vi "WILT Panel Dryer Details.vi"(0 "Dryer In":T4 {"Night Cycle Count" format="%04d"; "Day Cycle Count" format="%04d"}, 1 "FileName":path caption="Sample Datafilename", 9 "Test State":T2) -> (4 "Dryer Details Out":T3, 6 "New Filenames":bool, 8 "Updated":bool, 10 "Audit Alert Out":bool)   [LabVIEW 2016]
uses:
  Type Definitions/WILT Dryer.ctl
  Type Definitions/WILT Dryer Details.ctl
  Type Definitions/WILT Agilent Channel Definition.ctl
  Type Definitions/WILT DAQ Data.ctl
  Type Definitions/WILT Dryer Test State.ctl
  Globals/Globals Wilt.vi
panel:
  in  "Audit Alert Button":bool
  in  "Return":bool
  out "Time":dbl[](array[numeric])
  out "Cycle Count":dbl[](array[numeric])
  in  "Tab Control":T1(tab)
  out "Dryer Details":T3
  out "Total Cycle Count":i32
  out "Station Number":string
  out "Status Color":u32(colorbox)
  out "Bad Com Count":i32
  out "Com Port":u8
  out "Boolean":bool
  out "Audit Alert":bool
  out "Sample Plot":cluster{dbl[], dbl[]}[](graph)
  out "Current Cycle Count":dbl
  out "I(L1),I(L2),Trmb,V.V2":dbl[][](array[numeric])
  out "Cycle Count 2":dbl[](array[numeric])
  out "Completion time":dbl[](array[numeric])
  out "L1max":dbl[](array[numeric])
  out "L2max":dbl[](array[numeric])
  out "Tmax":dbl[](array[numeric])
  out "History Plot":cluster{dbl, dbl}[](graph)
  out "Serial Com Array":cluster{dbl, string}[](array[cluster]) {"?" format="%<%H:%M:%S>t"}
  out "Voltage 2":dbl[](array[numeric])
  out "Voltage":dbl[](array[numeric])
  out "Trmb":dbl[](array[numeric])
  out "L2":dbl[](array[numeric])
  out "L1":dbl[](array[numeric])
  out "Sample Record":string[][](array[string])
  out "all rows":string[][](array[string])
  in  "Read Sample Record(t, CC, Tc, \nASCII, Status, L1,L2,Trmb,V{,V2,SW} )":string[][](array[string])
  in  "Update":bool
  # "Day"
  # "Night"
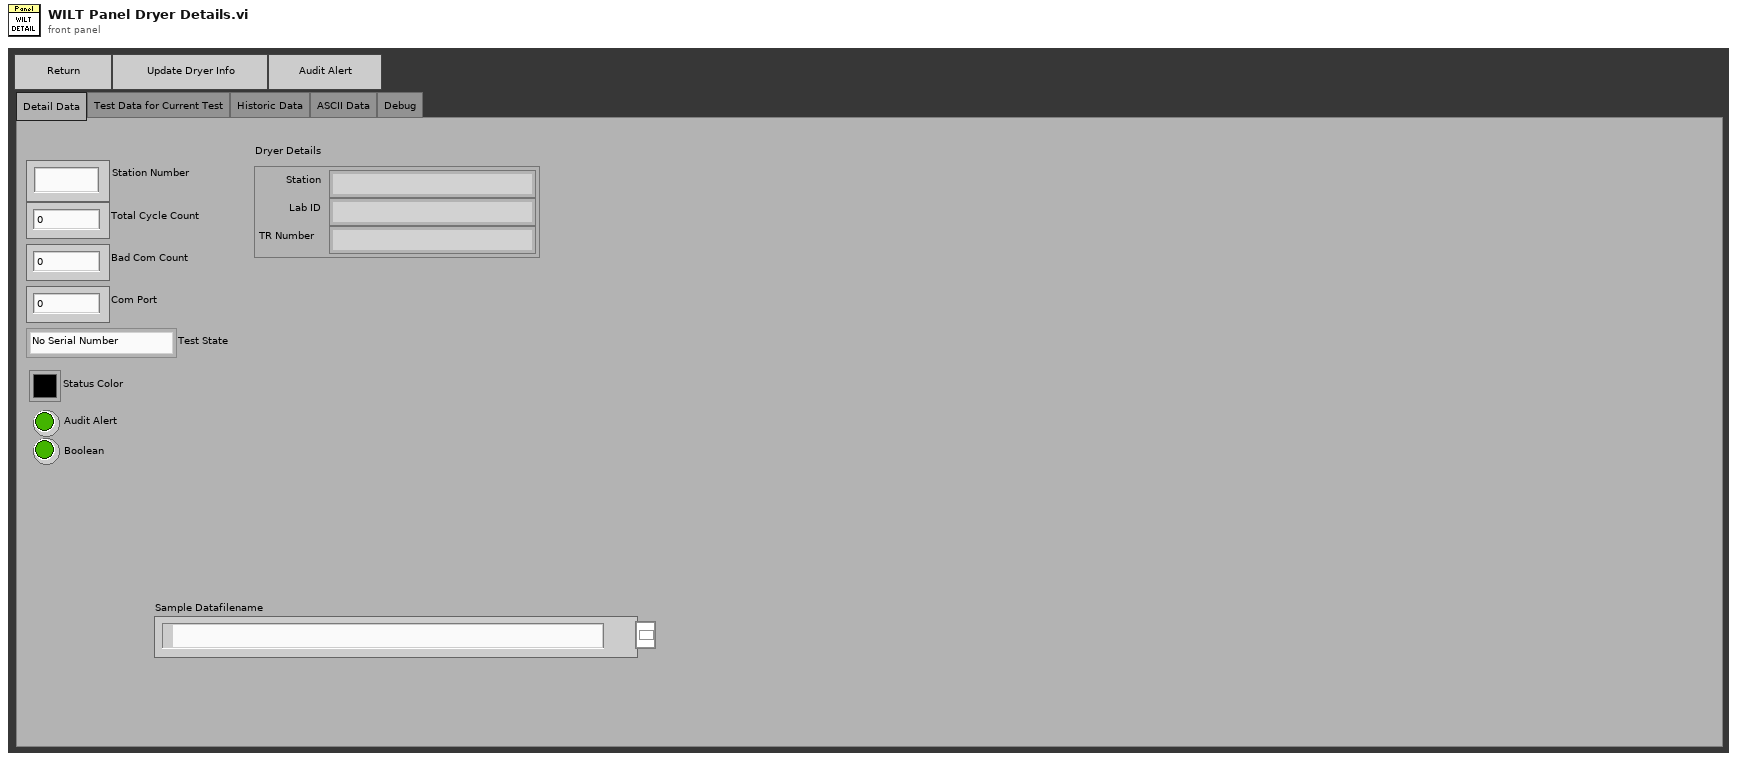
[diagram p1: front panel]
types:
  T1 = enum32{"Detail Data", "Test Data for Current Test", "Historic Data", "ASCII Data", "Debug"}
  T2 = typedef "WILT Dryer Test State.ctl" = enum16{"No Serial Number", "Waiting for Dryer To Start", "Drying Clothes", "Water Injection 1 (On)", "Water Injection 1 Timer", "Water Injection 1 (Off)", "Pause Dryer", "Sending Start Stop CMD", "Pause Dryer 2", "Sending Start Stop CMD 2", "Drying Clothes 2", "Water Injection 2 (On)", "Water Injection 2 Timer", "Water Injection 2 (Off)", "Drying Clothes 3", "Cooling Down", "Sending Start Stop CMD 3", "Increment Cycle"}
  T3 = typedef "WILT Dryer Details.ctl" = cluster{"Station":string, "Lab ID":string, "TR Number":string}
  T4 = typedef "WILT Dryer.ctl" = cluster{"Lab ID":string, "Day Cycle Count":i32, "Station Label":string, "Dryer Details":T3, "Status Color":u32, "Invisible Button":bool, "Night Cycle Count":i32, "Station Index":i32, "Cycle Index":string, "Audit Alert":bool, "Agilent Channel Definition":T5, "DAQ Data":T6}
  T5 = typedef "WILT Agilent Channel Definition.ctl" = cluster{"Channel":string, "Station":string, "Label":string, "Agilent Station":string, "Data":dbl}
  T6 = typedef "WILT DAQ Data.ctl" = cluster{"L1 Current":dbl, "L2 Current":dbl, "Temperature  Deg F (TC)":dbl, "Volts":dbl, "Volts (208)":dbl, "SW (208)":dbl}
  T7 = enum16{"Read 2D Array", "Write 2D Array", "Write/Append 1D Array"}
  T8 = cluster{"FileName":path, "New File Info":bool, "Dryer In":T4, "Read Sample Record(t, CC, Tc, \nASCII, Status, L1,L2,Trmb,V{,V2,SW} )":string[][], "Audit Alert":bool, "Updated":bool}
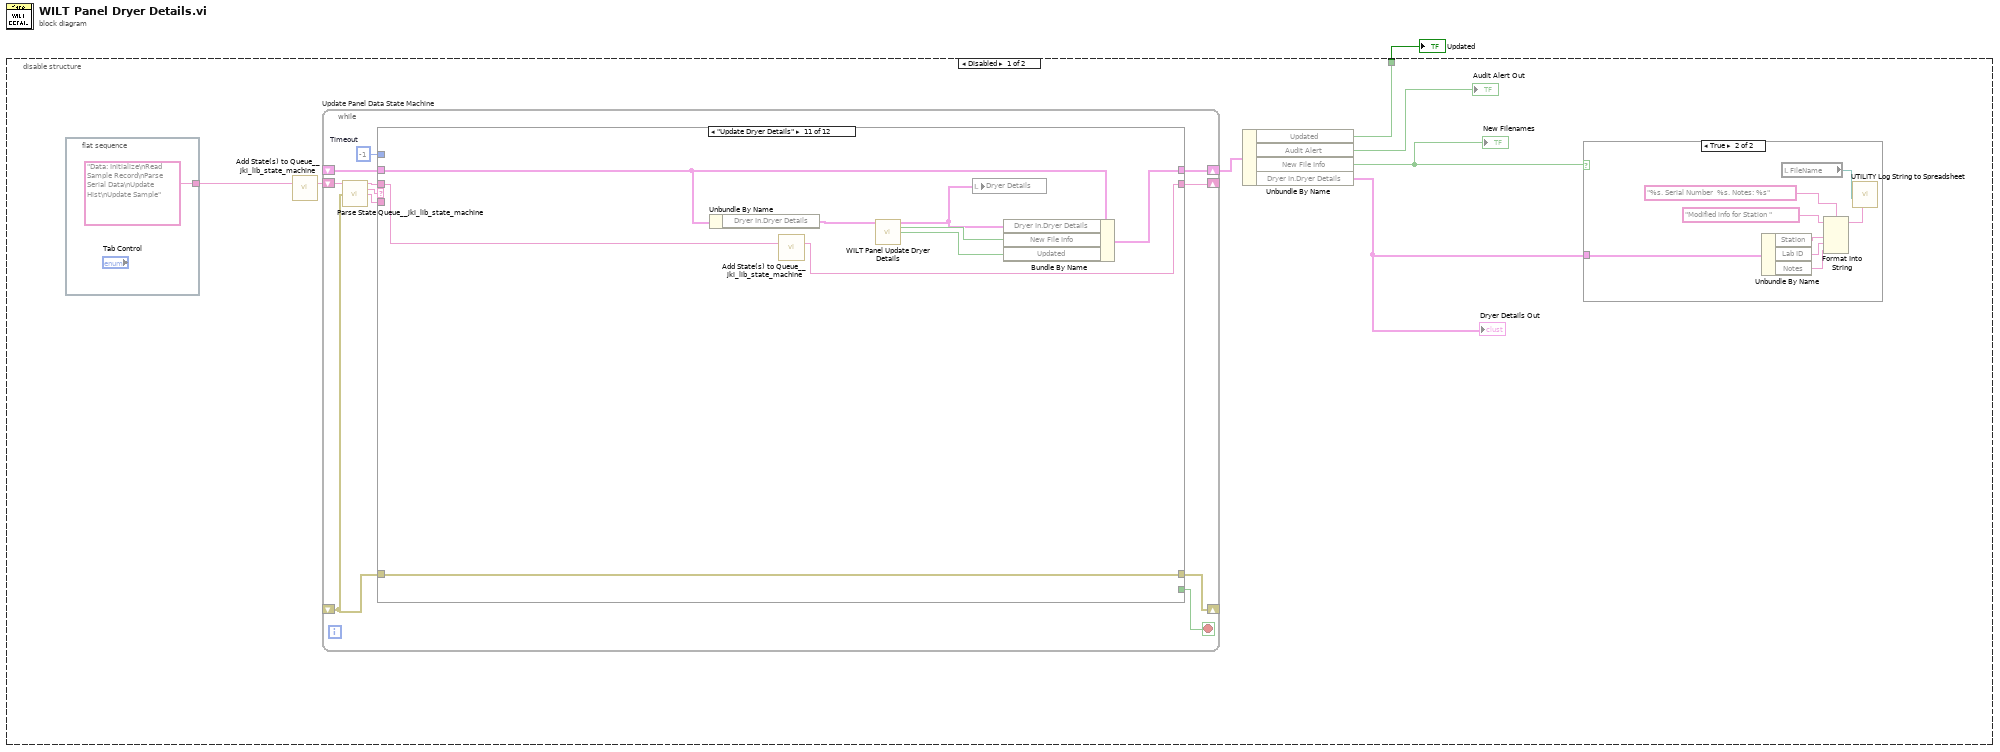
[diagram p0: block diagram]
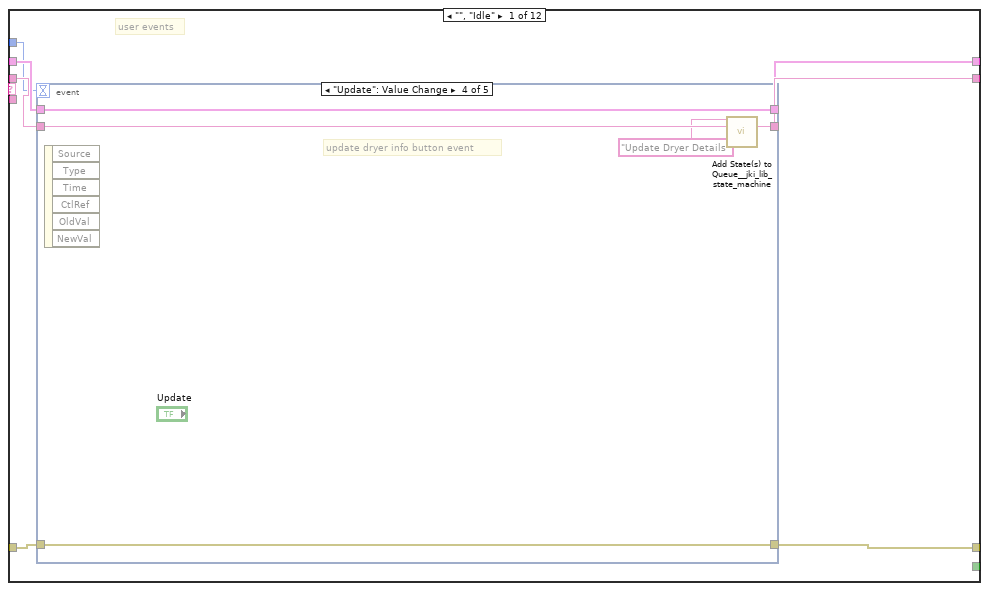
[diagram p2: hidden frame]
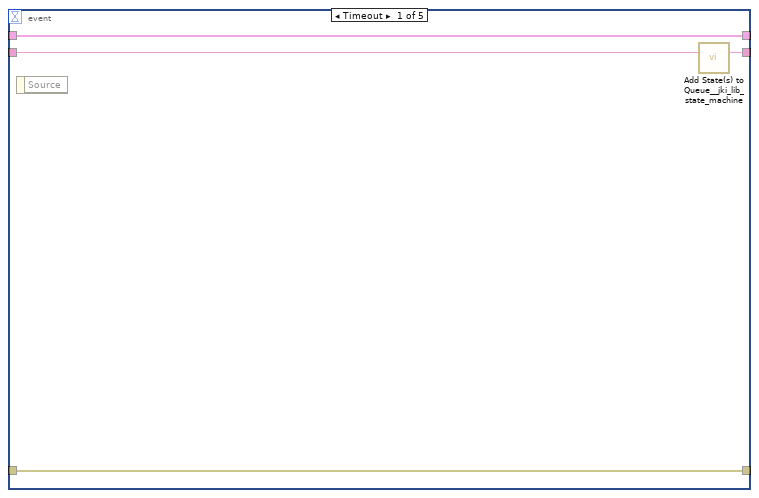
[diagram p3: hidden frame]
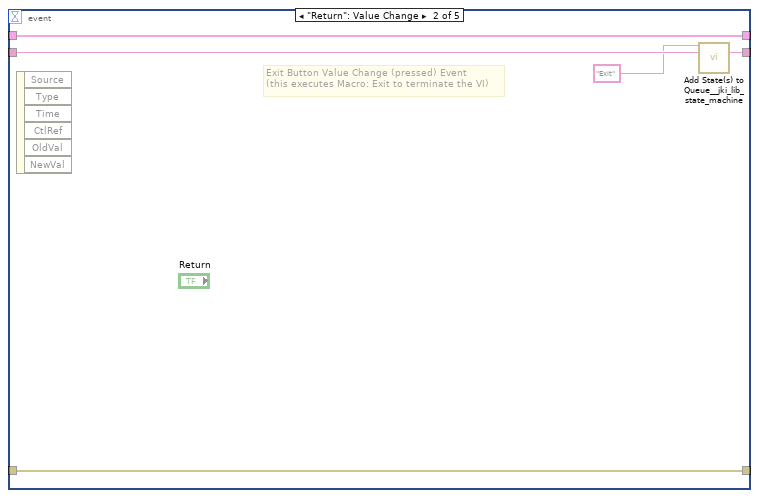
[diagram p4: hidden frame]
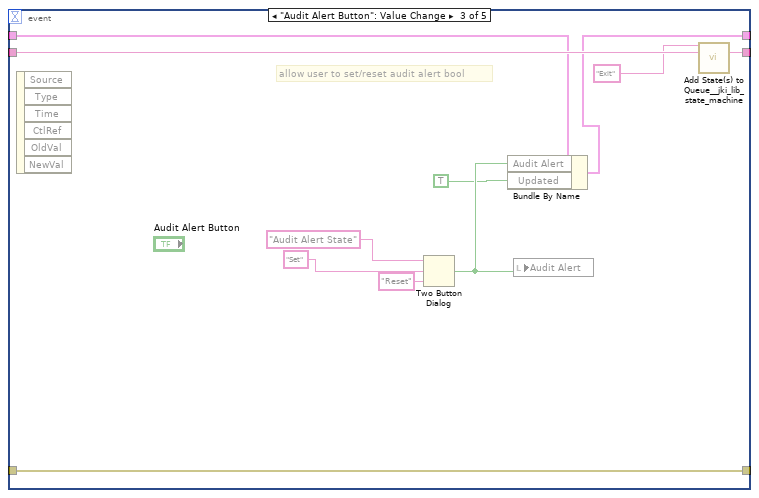
[diagram p5: hidden frame]
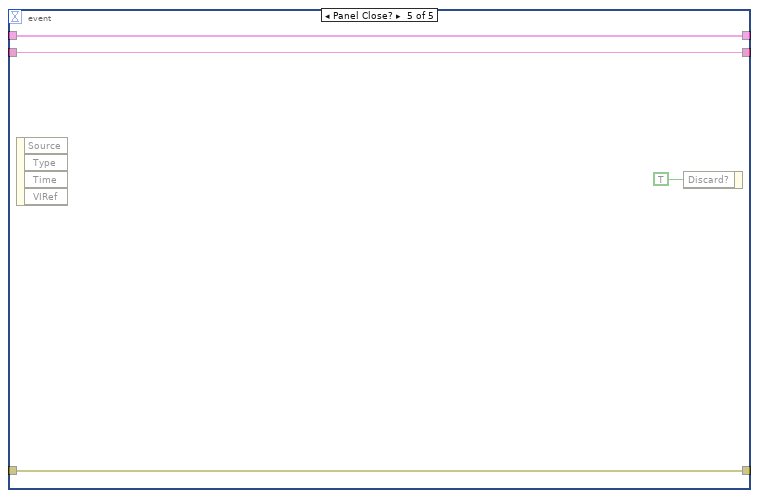
[diagram p6: hidden frame]
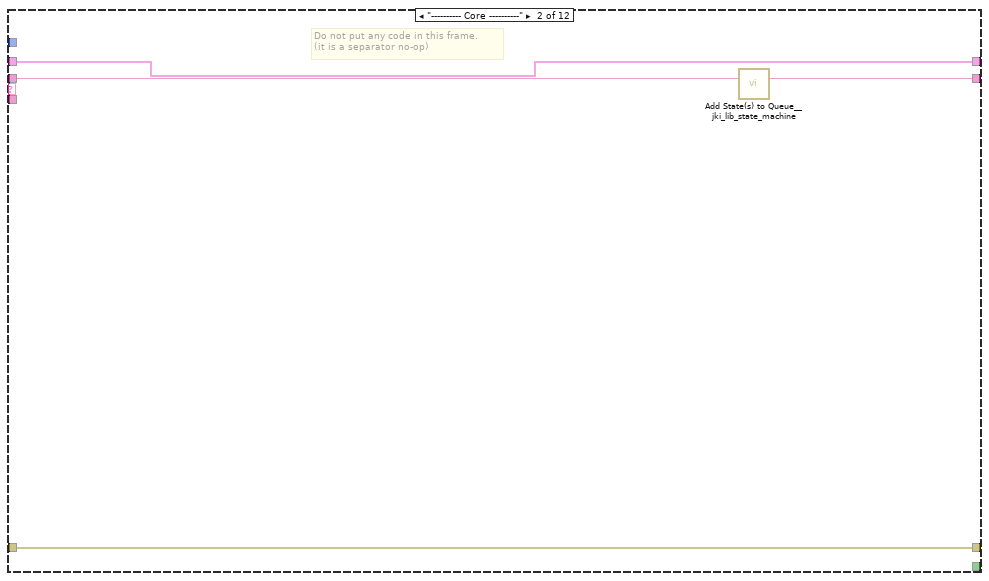
[diagram p7: hidden frame]
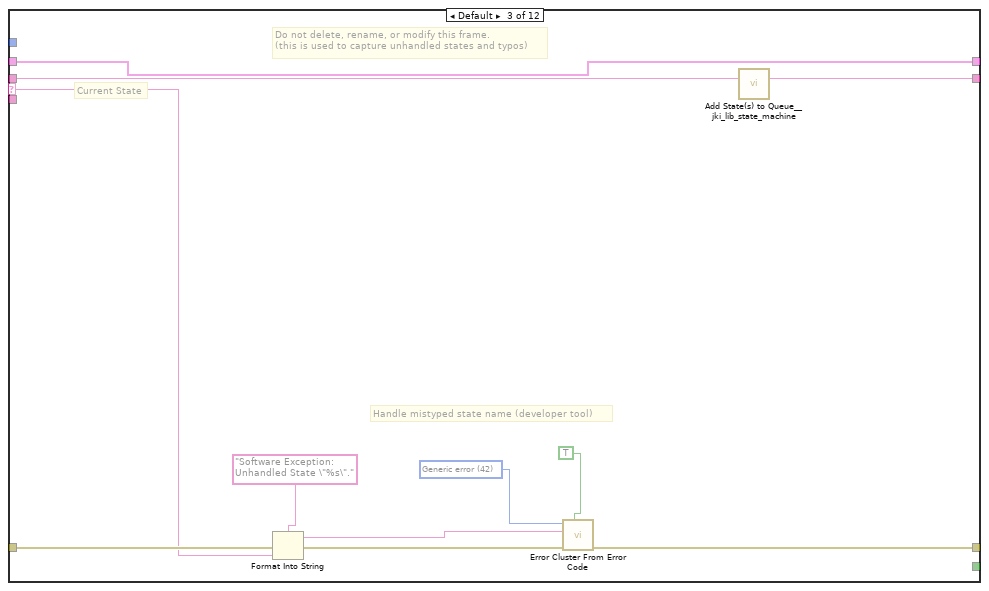
[diagram p8: hidden frame]
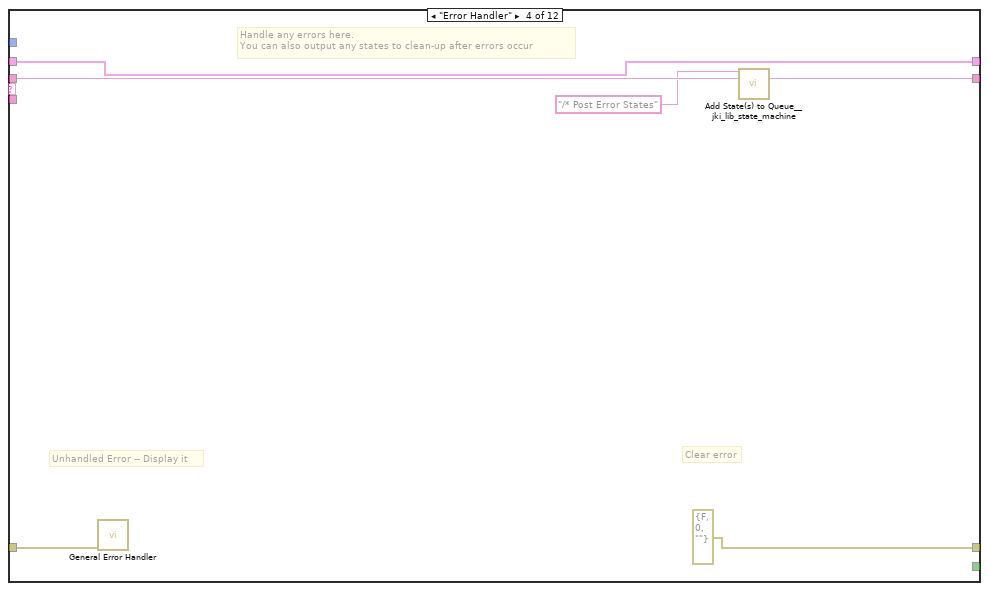
[diagram p9: hidden frame]
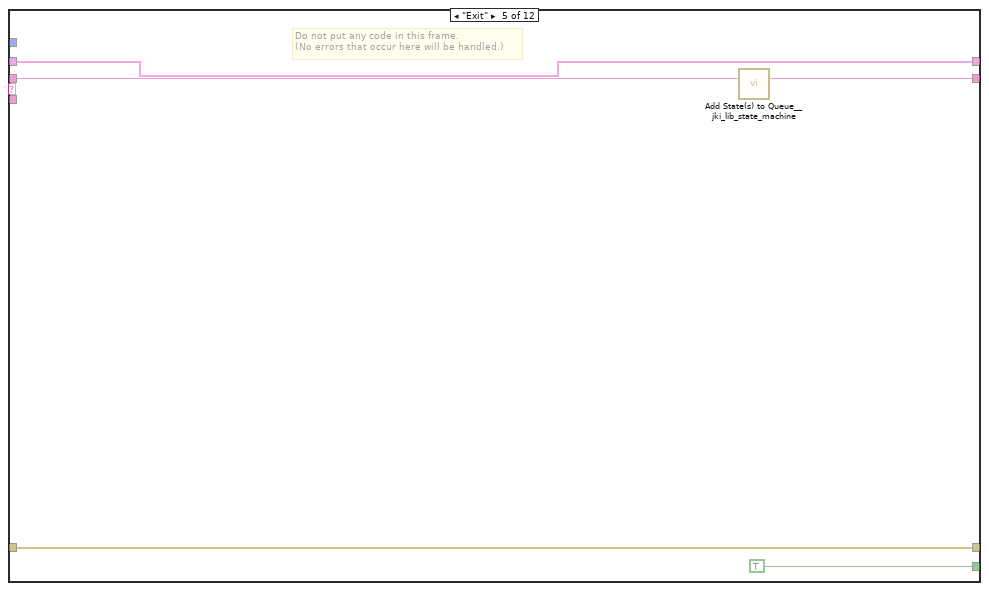
[diagram p10: hidden frame]
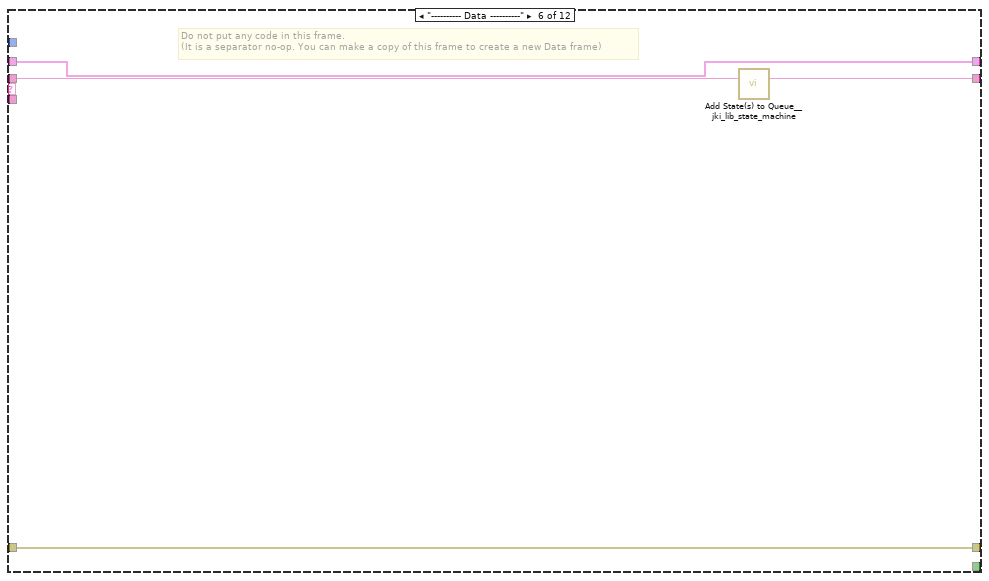
[diagram p11: hidden frame]
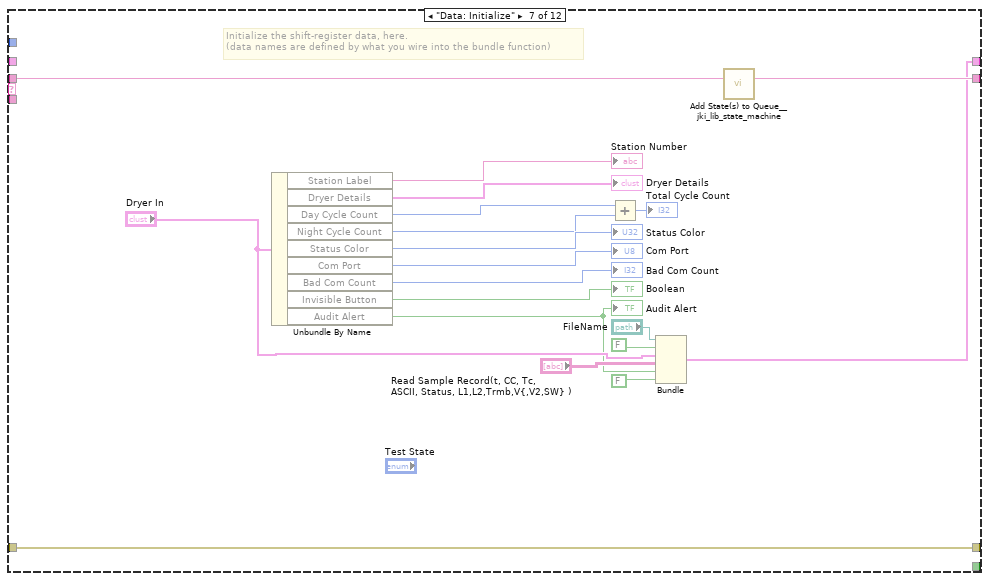
[diagram p12: hidden frame]
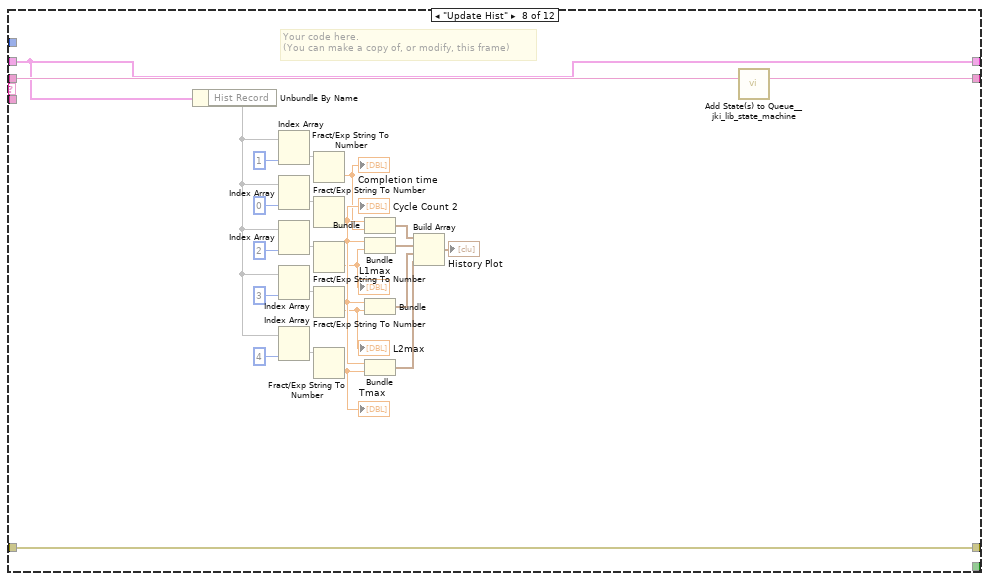
[diagram p13: hidden frame]
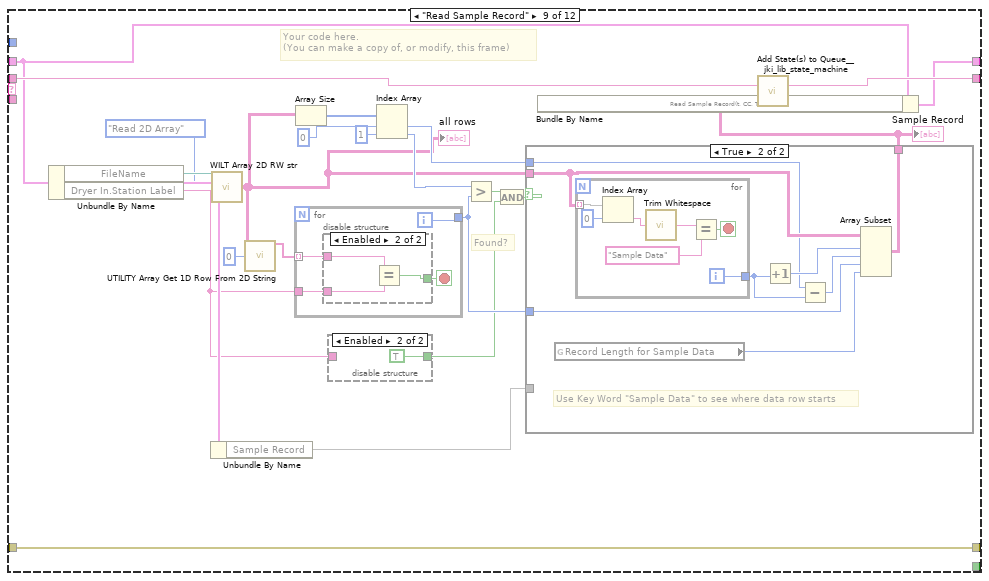
[diagram p14: hidden frame]
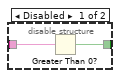
[diagram p15: hidden frame]
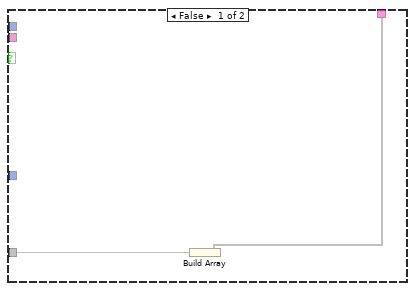
[diagram p16: hidden frame]
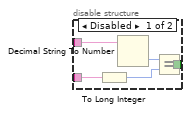
[diagram p17: hidden frame]
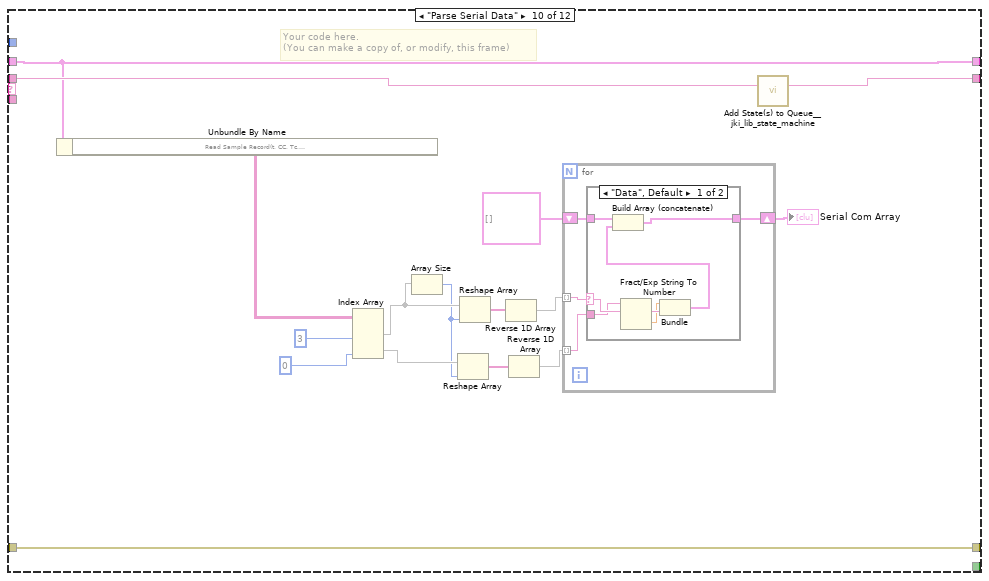
[diagram p18: hidden frame]
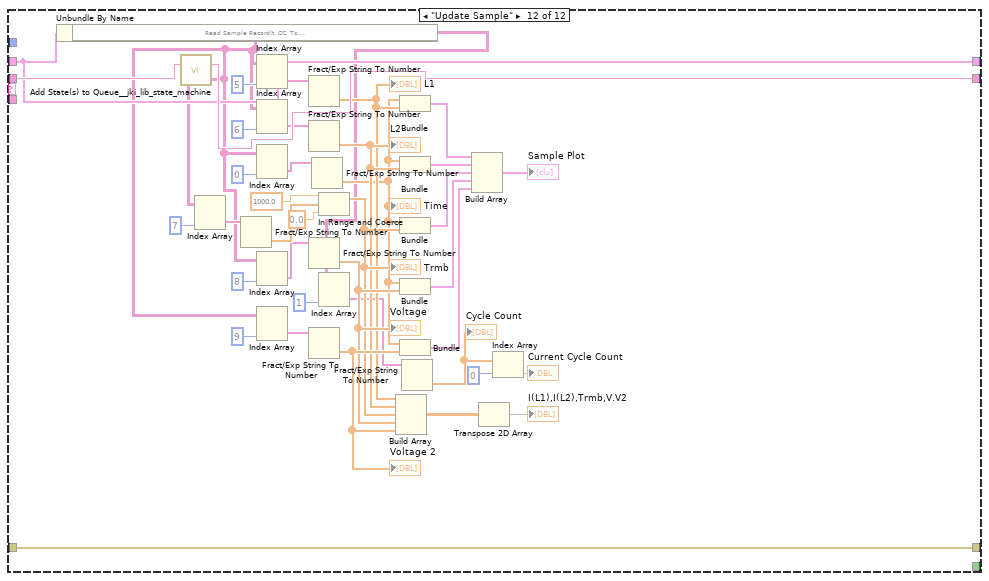
[diagram p20: hidden frame]
diagram:
  n1 = disable-structure shown="Disabled" {
    disable-tunnel: [w2 _] -> w1
    frame Disabled {
      n2 = flat-sequence {
        tunnel: ["Data: Initialize\nRead Sample Record\nParse Serial Data\nUpdate Hist\nUpdate Sample"] -> w7
        frame #0 {
        }
      }
      n3 = call <vilib>:"Add State(s) to Queue__jki_lib_state_machine.vi"("State(s) in (\"\")"=w7) -> ("States Out"=w8:string)  [unwired: 14 in]
      n4 = while "Update Panel Data State Machine" {
        shift-right: [w13] -> w6
        shift-left: _ -> [w12]
        shift-right: [w16] -> _
        shift-left: _ -> [w10]
        shift-right: [w15] -> _
        shift-left: w8 -> [w17]
        stop <- w14 stop-if-true
        w11 = -1  # Timeout
        n5 = call <vilib>:"Parse State Queue__jki_lib_state_machine.vi"("State Queue"=w17, "Error In (no error)"=w10) -> ("Remaining States"=w19:string, "Current State"=w20:string, "Arguments"=w18:string)  [unwired: 11 in]
        n6 = case shown="\"Update Dryer Details\"" w20 {
          selector: w20 -> [_ _ w61 _ _ _ _ _ _ _ _ _]
          tunnel: w19 -> [w27 w60 w65 w77 w82 w86 w105 w130 w152 w200 w220 w259]
          tunnel: w18 -> [_ _ _ _ _ _ _ _ _ _ _ _]
          tunnel: w12 -> [w25 w57 w63 w74 w80 w83 _ w107 w146 w197 w216 w222]
          tunnel: [w24 w58 w67 errorcluster {"status"=FALSE, "code"=0, "source"=""} ("error out") w79 w84 w102 w128 w150 w198 w218 w257] -> w16
          tunnel: w10 -> [w23 w58 w66 w73 w79 w84 w102 w128 w150 w198 w218 w257]
          tunnel: [w26 w59 w64 w76 w81 w85 w104 w129 w151 w199 w219 w258] -> w15
          tunnel: [_ _ _ _ TRUE _ _ _ _ _ _ _] -> w14
          tunnel: [w22 w57 w63 w74 w80 w83 w103 w107 w145 w197 w215 w222] -> w13
          tunnel: w11 -> [w21 _ _ _ _ _ _ _ _ _ _ _]
          frame "", "Idle" {
            # "user events"
            n7 = event shown="[3] \"Update\": Value Change" {
              selector: _ -> [_ _ _ _ _]
              dyn-events: _ -> [_ _ _ _ _]
              timeout: w21 -> [_ _ _ _ _]
              tunnel: w27 -> [w31 w36 w47 w52 w55]
              tunnel: [w30 w35 w46 w51 w55] -> w26
              tunnel: w25 -> [w28 w33 w40 w49 w56]
              tunnel: [w29 w34 w45 w50 w53] -> w24
              tunnel: w23 -> [w29 w34 w45 w50 w53]
              tunnel: [w28 w33 w39 w49 w56] -> w22
              event Timeout {
                n8 = event-data() -> ()  [unwired: 1 in, 1 out]
                n9 = call <vilib>:"Add State(s) to Queue__jki_lib_state_machine.vi"("State(s) in (\"\")"=w31) -> ("States Out"=w30:string)  [unwired: 14 in]
              }
              event "Return": Value Change {
                # "Exit Button Value Change (pressed) Event\n(this executes Macro: Exit to terminate the VI)"
                n10 = event-data() -> ()  [unwired: 1 in, 6 out]
                n11 = call <vilib>:"Add State(s) to Queue__jki_lib_state_machine.vi"("State(s) in Front (\"\")"="Exit", "State(s) in (\"\")"=w36) -> ("States Out"=w35:string)  [unwired: 13 in]
              }
              event "Audit Alert Button": Value Change {
                # "allow user to set/reset audit alert bool"
                n12 = event-data() -> ()  [unwired: 1 in, 6 out]
                n13 = Two Button Dialog(message="Audit Alert State", 1:"Reset" ("F button name (\"Cancel\")"), 2:"Set" ("T button name (\"OK\")")) -> (T button?=w38:bool)
                n14 = Bundle By Name(cluster=w40, "Audit Alert"=w38, "Updated"=TRUE) -> (w39:T8)
                n15 = local write "Audit Alert"(w38) -> ()
                n16 = call <vilib>:"Add State(s) to Queue__jki_lib_state_machine.vi"("State(s) in Front (\"\")"="Exit", "State(s) in (\"\")"=w47) -> ("States Out"=w46:string)  [unwired: 13 in]
              }
              event "Update": Value Change {
                # "update dryer info button event"
                n17 = event-data() -> ()  [unwired: 1 in, 6 out]
                n18 = call <vilib>:"Add State(s) to Queue__jki_lib_state_machine.vi"("State(s) in Front (\"\")"="Update Dryer Details", "State(s) in (\"\")"=w52) -> ("States Out"=w51:string)  [unwired: 13 in]
              }
              event Panel Close? {
                n19 = event-data() -> ()  [unwired: 1 in, 4 out]
                n20 = event-data("Discard?"=TRUE) -> ()  [unwired: 1 in, 1 out]
              }
            }
          }
          frame "---------- Core ----------" {
            # "Do not put any code in this frame.\n(it is a separator no-op)"
            n21 = call <vilib>:"Add State(s) to Queue__jki_lib_state_machine.vi"("State(s) in (\"\")"=w60) -> ("States Out"=w59:string)  [unwired: 14 in]
          }
          frame Default {
            w70 = 42 items=["No error", "Argument error", "Memory is full", "Out of zone", "End of file", "File already open", "Generic file I/O error", "File not found", "File permission error", "Disk is full", "Duplicate path", "Too many files open", "System feature not enabled", "Resource file not found", "Cannot add resource", "Resource not found", "Image not found", "Image memory error", "Pen does not exist", "Config type invalid", "Config token not found", "Config parse error", "Config memory error", "Bad external code format", "Bad external code offset", "External code not present", "Null window", "Destroy window error", "Null menu", "Print aborted", "Bad print record", "Print driver error", "Windows error during printing", "Memory error during printing", "Print dialog error", "Generic print error", "Invalid device refnum", "Device not found", "Device parameter error", "Device unit error", "Cannot open device", "Device call aborted", "Generic error", "Cancelled by user", "Object ID too low", "Object ID too high", "Object not in heap", "Unknown heap", "Unknown object (invalid DefProc)", "Unknown object (DefProc not in table)", "Message out of range", "Invalid (null) method", "Unknown message", "Manager call not supported", "Bad address", "Network operation in progress", "Network operation timed out", "Connection is busy", "Network attribute not supported", "Network error", "Address in use", "System out of memory", "Connection aborted", "Connection refused", "Not connected", "Already connected", "Connection closed", "Initialization error (interapplication manager)", "Bad occurrence", "Wait on unbound occurrence handler", "Occurrence queue overflow", "Datalog type conflict", "Unused", "Unrecognized type (interapplication manager)", "Memory corrupt", "Failed to make temporary DLL", "Old CIN version", "Drag socket not found", "Failed to load drop-object", "Failed to register OLE object", "Failed to release OLE object", "Format specifier type mismatch", "Unknown format specifier", "Too few format specifiers", "Too many format specifiers", "Scan failed", "Newer CIN version", "Error converting to variant", "Runtime menu error", "Password tampered", "Variant attribute not found", "Incompatible variant data type", "Event data is not available", "Event Store is not present", "Occurrence is not found", "Event Queue is not created", "Event info is not available", "Refnum passed is NULL", "Error retrieving Class GUID", "Error retrieving CoClass GUID", "Error retrieving TypeLib GUID.", "Bad built application magic bytes.", "Specific driver is different from the specific driver associated with the Logical Name.", "There is no session opened to the class driver.", "Max Error", "MAX - Error with config objects", "MAX - Error loading configuration", "MAX - Group not supported"]
            # "Current State"
            # "Do not delete, rename, or modify this frame.\n(this is used to capture unhandled states and typos)"
            # "Handle mistyped state name (developer tool)"
            n22 = Format Into String(format string="Software Exception: Unhandled State \"%s\"." ("message"), error in=w66, w61) -> (resulting string=w69:string, error out=w68:errorcluster)  [unwired: 1 in]
            n23 = call <vilib>:"Error Cluster From Error Code.vi"("show call chain? (False)"=TRUE, "error in (no error)"=w68, "error message (\"\")"=w69, "error code (0)"=w70) -> ("error out"=w67:errorcluster)  [unwired: 5 in]
            n24 = call <vilib>:"Add State(s) to Queue__jki_lib_state_machine.vi"("State(s) in (\"\")"=w65) -> ("States Out"=w64:string)  [unwired: 14 in]
          }
          frame "Error Handler" {
            # "Unhandled Error -- Display it"
            # "Handle any errors here.\nYou can also output any states to clean-up after errors occur"
            # "Clear error"
            n25 = call <vilib>:"General Error Handler.vi"("error in (no error)"=w73) -> ()  [unwired: 10 in, 5 out]
            n26 = call <vilib>:"Add State(s) to Queue__jki_lib_state_machine.vi"("State(s) in Front (\"\")"="/* Post Error States", "State(s) in (\"\")"=w77) -> ("States Out"=w76:string)  [unwired: 13 in]
          }
          frame "Exit" {
            # "Do not put any code in this frame.\n(No errors that occur here will be handled.)"
            n27 = call <vilib>:"Add State(s) to Queue__jki_lib_state_machine.vi"("State(s) in (\"\")"=w82) -> ("States Out"=w81:string)  [unwired: 14 in]
          }
          frame "---------- Data ----------" {
            # "Do not put any code in this frame.\n(It is a separator no-op. You can make a copy of this frame to create a new Data frame)"
            n28 = call <vilib>:"Add State(s) to Queue__jki_lib_state_machine.vi"("State(s) in (\"\")"=w86) -> ("States Out"=w85:string)  [unwired: 14 in]
          }
          frame "Data: Initialize" {
            # "Initialize the shift-register data, here.\n(data names are defined by what you wire into the bundle function)"
            n29 = Unbundle By Name("Dryer In") -> ("Station Label"=→"Station Number":string, "Dryer Details"=→"Dryer Details":T3, "Day Cycle Count"=w91:i32, "Night Cycle Count"=w90:i32, "Status Color"=→"Status Color":u32, "Com Port"=→"Com Port":u8, "Bad Com Count"=→"Bad Com Count":i32, "Invisible Button"=→"Boolean":bool, "Audit Alert"=w88:bool)
            "Audit Alert" <- w88
            n30 = Add(x=w91, y=w90) -> (x+y=→"Total Cycle Count":i32)
            n31 = Bundle("FileName"="FileName", "New File Info"=FALSE, "Dryer In"="Dryer In", "Read Sample Record(t, CC, Tc, \nASCII, Status, L1,L2,Trmb,V{,V2,SW} )"="Read Sample Record(t, CC, Tc, \nASCII, Status, L1,L2,Trmb,V{,V2,SW} )", "Audit Alert"=w88, "Updated"=FALSE) -> (w103:T8)  [unwired: 1 in]
            n32 = call <vilib>:"Add State(s) to Queue__jki_lib_state_machine.vi"("State(s) in (\"\")"=w105) -> ("States Out"=w104:string)  [unwired: 14 in]
          }
          frame "Update Hist" {
            # "Your code here.\n(You can make a copy of, or modify, this frame)"
            n33 = Unbundle By Name(w107) -> ("Hist Record"=w106)
            n34 = Index Array(array=w106, index (col)=1 ("disabled index (col)")) -> (element=w110)  [unwired: 1 in]
            n35 = Index Array(array=w106, index (col)=0 ("disabled index (col)")) -> (element=w108)  [unwired: 1 in]
            n36 = Index Array(array=w106, index (col)=2 ("disabled index (col)")) -> (element=w111)  [unwired: 1 in]
            n37 = Index Array(array=w106, index (col)=3 ("disabled index (col)")) -> (element=w115)  [unwired: 1 in]
            n38 = Index Array(array=w106, index (col)=4 ("disabled index (col)")) -> (element=w124)  [unwired: 1 in]
            n39 = Fract/Exp String To Number(string=w110) -> (number=w116:dbl)  [unwired: 3 in, 1 out]
            "Completion time" <- w116
            n40 = Fract/Exp String To Number(string=w108) -> (number=w126:dbl)  [unwired: 3 in, 1 out]
            "Cycle Count 2" <- w126
            n41 = Fract/Exp String To Number(string=w111) -> (number=w117:dbl)  [unwired: 3 in, 1 out]
            "L1max" <- w117
            n42 = Fract/Exp String To Number(string=w115) -> (number=w118:dbl)  [unwired: 3 in, 1 out]
            "L2max" <- w118
            n43 = Fract/Exp String To Number(string=w124) -> (number=w125:dbl)  [unwired: 3 in, 1 out]
            "Tmax" <- w125
            n44 = Bundle(w126, w116) -> (w120:cluster{dbl, dbl})  [unwired: 1 out]
            n45 = Bundle(w126, w117) -> (w121:cluster{dbl, dbl})  [unwired: 1 out]
            n46 = Bundle(w126, w118) -> (w122:cluster{dbl, dbl})  [unwired: 1 out]
            n47 = Bundle(w126, w125) -> (w127:cluster{dbl, dbl})  [unwired: 1 out]
            n48 = Build Array(w120, w121, w122, w127) -> (→"History Plot":cluster{dbl, dbl}[])
            n49 = call <vilib>:"Add State(s) to Queue__jki_lib_state_machine.vi"("State(s) in (\"\")"=w130) -> ("States Out"=w129:string)  [unwired: 14 in]
          }
          frame "Read Sample Record" {
            # "Found?"
            # "Your code here.\n(You can make a copy of, or modify, this frame)"
            n50 = Unbundle By Name(w146) -> ("FileName"=w133:path, "Dryer In.Station Label"=w141:string)
            n51 = Unbundle By Name(w146) -> ("Sample Record"=w139)
            n52 = call "WILT Array 2D RW str.vi"("file path (dialog if empty)"=w133, "Write/Read"=T7."Read 2D Array") -> ("Read all rows"=w132:string[][])  [unwired: 13 in]
            "all rows" <- w132
            n53 = call "UTILITY Array Get 1D Row From 2D String.vi"("all rows"=w132, "row index"=0) -> ("row"=w136:string[])  [unwired: 13 in]
            n54 = for {
              tunnel: w136 -> [w176] mode=indexing
              tunnel: w141 -> [w175]
              tunnel: [w173] -> w147
              i -> [w173]
              stop <- w174 stop-if-true
              n55 = disable-structure shown="Enabled" {
                disable-tunnel: w176 -> [w181 w183]
                disable-tunnel: w175 -> [w179 w184]
                disable-tunnel: [w177 w182] -> w174
                frame Disabled {
                  n56 = To Long Integer(number=w179) -> (32bit integer=w178:i32)
                  n57 = Decimal String To Number(string=w181) -> (number=w180:i32)  [unwired: 2 in, 1 out]
                  n58 = Equal?(x=w180, y=w178) -> (x = y?=w177:bool)
                }
                frame Enabled {
                  n59 = Equal?(x=w183, y=w184) -> (x = y?=w182:bool)
                }
              }
            }
            n60 = Array Size(array=w132) -> (size(s)=w149:i32[])
            n61 = disable-structure shown="Enabled" {
              disable-tunnel: w141 -> [w154 _]
              disable-tunnel: [w153 TRUE] -> w140
              frame Disabled {
                n62 = Greater Than 0?(x=w154) -> (x > 0?=w153:bool)
              }
              frame Enabled {
              }
            }
            n63 = Index Array(array=w149, index #1=0 ("index"), index #2=1 ("index")) -> (element #1=w134:i32, element #2=w137:i32)
            n64 = Greater?(x=w137, y=w147) -> (0:w143:bool)
            n65 = And(x=w143, y=w140) -> (x .and. y?=w142:bool)
            n66 = case shown="True" w142 {
              tunnel: w132 -> [_ w164]
              tunnel: w147 -> [_ w163]
              tunnel: [w156 w162] -> w144
              tunnel: w139 -> [w157 _]
              tunnel: w134 -> [_ w159]
              frame False {
                n67 = Build Array(w157) -> (w156:void[])
              }
              frame True {
                # "Use Key Word \"Sample Data\" to see where data row starts"
                n68 = global read "Globals Wilt.vi" "Record Length for Sample Data"() -> (w161:i32)
                n69 = for {
                  tunnel: w164 -> [w172] mode=indexing
                  tunnel: [w169] -> w158
                  i -> [w169]
                  stop <- w168 stop-if-true
                  n70 = Index Array(array=w172, index=0) -> (element=w167:string)
                  n71 = call <vilib>:"Trim Whitespace.vi"("string"=w167) -> ("trimmed string"=w166:string)  [unwired: 1 in]
                  n72 = Equal?(x=w166, y="Sample Data") -> (x = y?=w168:bool)
                }
                n73 = Increment(x=w158) -> (x+1=w165:i32)
                n74 = Subtract(x=w159, y=w158) -> (x-y=w160:i32)
                n75 = Array Subset(array=w164, index (row)=w165, length (row)=w160, index (col)=w163, length (col)=w161) -> (w162:string[][])
              }
            }
            "Sample Record" <- w144
            n76 = Bundle By Name(cluster=w146, "Read Sample Record(t, CC, Tc, \nASCII, Status, L1,L2,Trmb,V{,V2,SW} )"=w144) -> (w145:T8)
            n77 = call <vilib>:"Add State(s) to Queue__jki_lib_state_machine.vi"("State(s) in (\"\")"=w152) -> ("States Out"=w151:string)  [unwired: 14 in]
          }
          frame "Parse Serial Data" {
            # "Your code here.\n(You can make a copy of, or modify, this frame)"
            n78 = Unbundle By Name(w197) -> ("Read Sample Record(t, CC, Tc, \nASCII, Status, L1,L2,Trmb,V{,V2,SW} )"=w187:string[][])
            n79 = Index Array(array=w187, index (col) #1=3 ("disabled index (col)"), index (col) #2=0 ("index (col)")) -> (element #1=w186:string[], element #2=w193:string[])  [unwired: 2 in]
            n80 = Array Size(array=w186) -> (size(s)=w185:i32)
            n81 = Reshape Array(w193, w185) -> (w192:string[])
            n82 = Reshape Array(w186, w185) -> (w195:string[])
            n83 = Reverse 1D Array(array=w195) -> (reversed array=w191:string[])
            n84 = Reverse 1D Array(array=w192) -> (reversed array=w190:string[])
            n85 = for {
              tunnel: w191 -> [w204] mode=indexing
              tunnel: w190 -> [w203] mode=indexing
              shift-right: [w202] -> w189
              shift-left: cluster{dbl, string}[] [] -> [w201]
              n86 = case shown="\"Data\", Default" w204 {
                selector: w204 -> [w210 _]
                tunnel: w203 -> [w209 _]
                tunnel: [w207 w211] -> w202
                tunnel: w201 -> [w206 w211]
                frame "Data", Default {
                  n87 = Fract/Exp String To Number(string=w209) -> (number=w205:dbl)  [unwired: 3 in, 1 out]
                  n88 = Bundle(w205, w210) -> (w208:cluster{dbl, string})  [unwired: 1 in]
                  n89 = Build Array (concatenate)(w206, w208) -> (w207:cluster{dbl, string}[])
                }
                frame "" {
                }
              }
            }
            "Serial Com Array" <- w189
            n90 = call <vilib>:"Add State(s) to Queue__jki_lib_state_machine.vi"("State(s) in (\"\")"=w200) -> ("States Out"=w199:string)  [unwired: 14 in]
          }
          frame "Update Dryer Details" {
            n91 = Unbundle By Name(w216) -> ("Dryer In.Dryer Details"=w217:T3)
            n92 = call <vilib>:"Add State(s) to Queue__jki_lib_state_machine.vi"("State(s) in (\"\")"=w220) -> ("States Out"=w219:string)  [unwired: 14 in]
            n93 = call "WILT Panel Update Dryer Details.vi"("Dryer Details In"=w217) -> ("Dryer Details Out"=w213:T3, "New Filenames"=w214:bool, "Updated"=w212:bool)  [unwired: 12 in]
            n94 = local write "Dryer Details"(w213) -> ()
            n95 = Bundle By Name(cluster=w216, "Dryer In.Dryer Details"=w213, "New File Info"=w214, "Updated"=w212) -> (w215:T8)
          }
          frame "Update Sample" {
            n96 = Unbundle By Name(w222) -> ("Read Sample Record(t, CC, Tc, \nASCII, Status, L1,L2,Trmb,V{,V2,SW} )"=w221:string[][])
            n97 = call <vilib>:"Add State(s) to Queue__jki_lib_state_machine.vi"("State(s) in (\"\")"=w259) -> ("States Out"=w258:string)  [unwired: 14 in]
            n98 = Index Array(array=w221, index (col)=7 ("disabled index (col)")) -> (element=w231:string[])  [unwired: 1 in]
            n99 = Fract/Exp String To Number(string=w231) -> (number=w247:dbl[])  [unwired: 3 in, 1 out]
            n100 = Index Array(array=w221, index (col)=5 ("disabled index (col)")) -> (element=w226:string[])  [unwired: 1 in]
            n101 = Index Array(array=w221, index (col)=6 ("disabled index (col)")) -> (element=w228:string[])  [unwired: 1 in]
            n102 = Index Array(array=w221, index (col)=0 ("disabled index (col)")) -> (element=w224:string[])  [unwired: 1 in]
            n103 = Index Array(array=w221, index (col)=8 ("disabled index (col)")) -> (element=w233:string[])  [unwired: 1 in]
            n104 = Index Array(array=w221, index (col)=9 ("disabled index (col)")) -> (element=w235:string[])  [unwired: 1 in]
            n105 = Fract/Exp String To Number(string=w226) -> (number=w250:dbl[])  [unwired: 3 in, 1 out]
            "L1" <- w250
            n106 = Fract/Exp String To Number(string=w228) -> (number=w251:dbl[])  [unwired: 3 in, 1 out]
            "L2" <- w251
            n107 = Fract/Exp String To Number(string=w233) -> (number=w253:dbl[])  [unwired: 3 in, 1 out]
            "Voltage" <- w253
            n108 = Fract/Exp String To Number(string=w235) -> (number=w254:dbl[])  [unwired: 3 in, 1 out]
            "Voltage 2" <- w254
            n109 = Fract/Exp String To Number(string=w224) -> (number=w237:dbl[])  [unwired: 3 in, 1 out]
            "Time" <- w237
            n110 = In Range and Coerce(upper limit=1000.0 ("String"), x=w247, lower limit=0.0 ("String")) -> (coerced(x)=w252:dbl[])  [unwired: 1 out]
            "Trmb" <- w252
            n111 = Index Array(array=w221, index (col)=1 ("disabled index (col)")) -> (element=w225:string[])  [unwired: 1 in]
            n112 = Build Array(w250, w251, w252, w253, w254) -> (w255:dbl[][])
            n113 = Bundle(w237, w250) -> (w239:cluster{dbl[], dbl[]})  [unwired: 1 out]
            n114 = Bundle(w237, w251) -> (w238:cluster{dbl[], dbl[]})  [unwired: 1 out]
            n115 = Bundle(w237, w252) -> (w240:cluster{dbl[], dbl[]})  [unwired: 1 out]
            n116 = Bundle(w237, w253) -> (w241:cluster{dbl[], dbl[]})  [unwired: 1 out]
            n117 = Bundle(w237, w254) -> (w242:cluster{dbl[], dbl[]})  [unwired: 1 out]
            n118 = Fract/Exp String To Number(string=w225) -> (number=w244:dbl[])  [unwired: 3 in, 1 out]
            "Cycle Count" <- w244
            n119 = Build Array(w239, w238, w240, w241, w242) -> (→"Sample Plot":cluster{dbl[], dbl[]}[])
            n120 = Transpose 2D Array(2D array=w255) -> (transposed array=→"I(L1),I(L2),Trmb,V.V2":dbl[][])
            n121 = Index Array(array=w244, index=0) -> (element=→"Current Cycle Count":dbl)
          }
        }
      }
      n122 = Unbundle By Name(w6) -> ("Updated"=w2:bool, "Audit Alert"=→"Audit Alert Out":bool, "New File Info"=w4:bool, "Dryer In.Dryer Details"=w5:T3)
      "Dryer Details Out" <- w5
      "New Filenames" <- w4
      n123 = case shown="True" w4 {
        tunnel: w5 -> [_ w266]
        frame False {
        }
        frame True {
          n124 = Unbundle By Name(w266) -> ("Station"=w265:string, "Lab ID"=w263:string, "Notes"=w262:string)
          n125 = local read "FileName"() -> (w260:path)
          n126 = Format Into String(format string="%s. Serial Number  %s. Notes: %s", initial string="Modified info for Station ", w265, w263, w262) -> (resulting string=w261:string)  [unwired: 1 in, 1 out]
          n127 = call "UTILITY Log String to Spreadsheet.vi"("String"=w261, "FileName"=w260) -> ()  [unwired: 9 in, 1 out]
        }
      }
    }
    frame Enabled {
    }
  }
  "Updated" <- w1
